vi "Pack JSON Message.vi"(8 "error in (no error)":errorcluster, 11 "Tcp Message":T1={"Command"="", "Data"=[], "Script ID"=0, "LabVIEW Server ID"="zxcvbnm,", "Python Message ID"=0}) -> (0 "error out":errorcluster, 3 "String":string)   [LabVIEW 2013, in "TS.lvlib"]
uses:
  TS.lvlib
  LabVIEW Python Connector Message.ctl
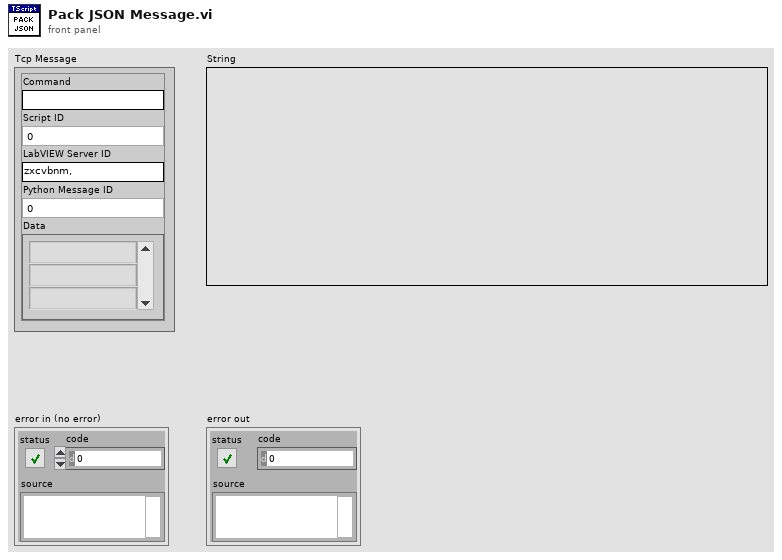
[diagram p1: front panel]
types:
  T1 = typedef "TS.lvlib/LabVIEW Python Connector Message.ctl" = cluster{"Command":string, "Data":string[], "Script ID":i64, "LabVIEW Server ID":string, "Python Message ID":i32}
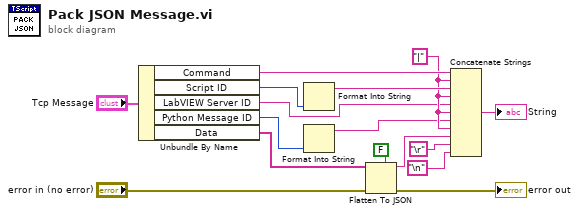
[diagram p0: block diagram]
diagram:
  w6 = "|"
  n1 = Unbundle By Name("Tcp Message") -> ("Command"=w14:string, "Script ID"=w15:i64, "LabVIEW Server ID"=w2:string, "Python Message ID"=w4:i32, "Data"=w1:string[])
  n2 = Format Into String(w15) -> (resulting string=w16:string)  [unwired: 3 in, 1 out]
  n3 = Format Into String(w4) -> (resulting string=w3:string)  [unwired: 3 in, 1 out]
  n4 = Flatten To JSON(enable LabVIEW extensions? (T)=FALSE, anything=w1, error in (no error)="error in (no error)") -> (JSON string=w5:string, 11:→"error out":errorcluster)
  n5 = Concatenate Strings(w14, w6, w16, w6, w2, w6, w3, w6, w5, "\r", "\n") -> (→"String":string)
